vi "Maze.vi"(10 "Status Notifier":refnum<notifier>, 11 "Submission LLB":path) -> (0 "error out":errorcluster, 2 "Test Summary":string, 3 "Score":T1)   [LabVIEW 2020]
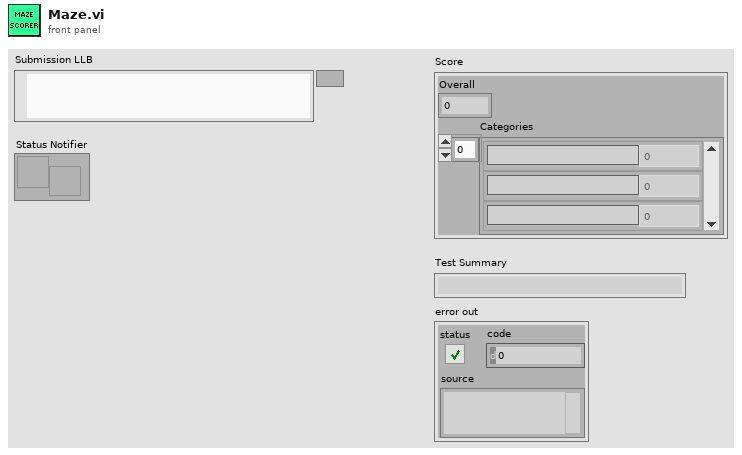
[diagram p1: front panel]
types:
  T1 = cluster{"Overall":dbl, "Categories":cluster{"Category":string, "Value":dbl}[]}
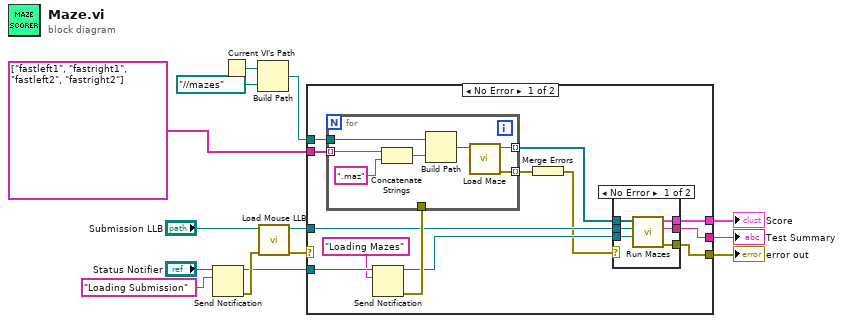
[diagram p0: block diagram]
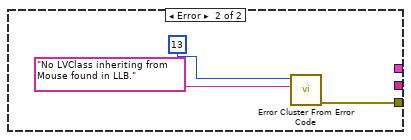
[diagram p3: hidden frame]
diagram:
  n1 = Send Notification(notification="Loading Submission", notifier="Status Notifier") -> (notifier out=w3:refnum<notifier>, error out=w11:errorcluster)  [unwired: 1 in]
  n2 = Current VI's Path() -> (path=w7:path)
  n3 = Build Path(base path=w7, name or relative path=path "../../mazes") -> (appended path=w4:path)
  n4 = call "Load Mouse LLB.vi"("error in (no error)"=w11, "Mouse LLB"="Submission LLB") -> ("error out"=w9:errorcluster, "Mouse"=w10:refnum<class "Mouse.lvclass">)  [unwired: 7 in, 1 out]
  n5 = case shown="No Error" w9 {
    tunnel: w10 -> [w21 _]
    tunnel: [w17 w42] -> w8
    tunnel: string[] ["fastleft1", "fastright1", "fastleft2", "fastright2"] -> [w27 _]
    tunnel: w4 -> [w26 _]
    tunnel: w3 -> [w25 _]
    tunnel: [w19 _] -> w2
    tunnel: [w18 _] -> w1
    frame No Error {
      n6 = Send Notification(notification="Loading Mazes", notifier=w25) -> (notifier out=w20:refnum<notifier>, error out=w23:errorcluster)  [unwired: 1 in]
      n7 = for {
        tunnel: w27 -> [w41] mode=indexing
        tunnel: w26 -> [w39]
        tunnel: [w36] -> w22 mode=indexing
        tunnel: w23 -> [_]
        tunnel: [w35] -> w16 mode=indexing
        n8 = Concatenate Strings(w41, ".maz" ("string")) -> (w38:string)
        n9 = Build Path(base path=w39, name or relative path=w38) -> (appended path=w37:path)
        n10 = call "Load Maze.vi"("Maze File Path (*.maz)"=w37) -> ("error out"=w35:errorcluster, "Maze"=w36:refnum<class "Maze.lvclass">)  [unwired: 9 in]
      }
      n11 = Merge Errors(w16) -> (w15:errorcluster)
      n12 = case shown="No Error" w15 {
        selector: w15 -> [_ w34]
        tunnel: w22 -> [w33 _]
        tunnel: w21 -> [w32 _]
        tunnel: w20 -> [w31 _]
        tunnel: [w30 _] -> w19
        tunnel: [w29 _] -> w18
        tunnel: [w28 w34] -> w17
        frame No Error {
          n13 = call "Run Mazes.vi"("Status Notifier"=w31, "Mouse"=w32, "Mazes"=w33) -> ("error out"=w28:errorcluster, "Test Summary"=w29:string, "Score"=w30:T1)  [unwired: 6 in]
        }
        frame Error {
        }
      }
    }
    frame Error {
      n14 = call <vilib>:"Error Cluster From Error Code.vi"("error message (\"\")"="No LVClass inheriting from Mouse found in LLB." ("error message (\"\")"), "error code (0)"=13) -> ("error out"=w42:errorcluster)  [unwired: 7 in]
    }
  }
  "Score" <- w2
  "Test Summary" <- w1
  "error out" <- w8
